vi "Ear control.vi"(11 "Toggle Ears":bool) -> ()   [LabVIEW 2012]
uses:
  <vilib>/Rock Robotics/WPI/Solenoid/WPI_SolenoidValue.ctl
  <vilib>/Rock Robotics/WPI/Solenoid/WPI_SolenoidGetEnum.vi
  <vilib>/Rock Robotics/WPI/Solenoid/WPI_SolenoidSetEnum.vi
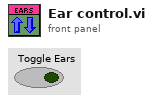
[diagram p1: front panel]
types:
  T1 = typedef "WPI_SolenoidValue.ctl" = enum16{"Off", "On", "Forward", "Reverse"}
  T2 = typedef "WPI_SolenoidDevRef.ctl" = cluster{"DevStatus":errorcluster, "Solenoid Module":T3, "Forward Solenoid Channel":T4, "Reverse Solenoid Channel":T4}
  T3 = typedef "FPGA_TypedefSolenoidModule.ctl" = enum16{"Solenoid Module 1", "Solenoid Module 2"}
  T4 = typedef "WPI_SolenoidChannel.ctl" = enum8{"Solenoid 1", "Solenoid 2", "Solenoid 3", "Solenoid 4", "Solenoid 5", "Solenoid 6", "Solenoid 7", "Solenoid 8", "Invalid"}
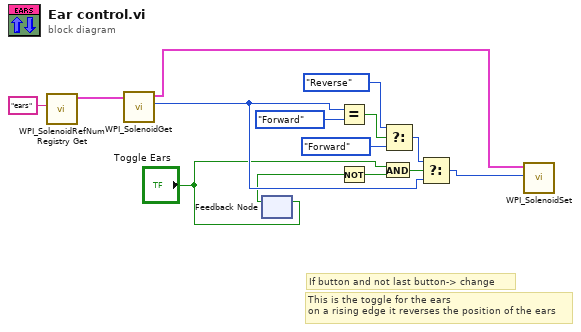
[diagram p0: block diagram]
diagram:
  # "If button and not last button-> change"
  # "This is the toggle for the ears\non a rising edge it reverses the position of the ears"
  n1 = call <vilib>:"WPI_SolenoidRefNum Registry Get.vi"("refnum name"="ears") -> ("SolenoidDevRef"=w7:T2)  [unwired: 9 in, 1 out]
  n2 = call-poly <vilib>:"WPI_SolenoidGet.vi"("SolenoidDevRef"=w7) -> ("Value"=w10:T1, "SolenoidDevRef"=w1:T2)  [unwired: 8 in, 1 out]
  n3 = feedback #1() -> (w5:bool)  [unwired: 1 in]
  n4 = feedback-in #1("Toggle Ears") -> ()
  n5 = Equal?(x=w10, y=WPI_SolenoidValue."Forward" ("s? t:f")) -> (x = y?=w11:bool)
  n6 = Not(x=w5) -> (.not. x?=w3:bool)
  n7 = And(x="Toggle Ears", y=w3) -> (x .and. y?=w6:bool)
  n8 = Select(t=WPI_SolenoidValue."Reverse" ("s? t:f"), s=w11, f=WPI_SolenoidValue."Forward" ("s? t:f")) -> (s? t:f=w14:T1)
  n9 = Select(t=w14, s=w6, f=w10) -> (s? t:f=w2:T1)
  n10 = call-poly <vilib>:"WPI_SolenoidSet.vi"("Value"=w2, "SolenoidDevRef"=w1) -> ()  [unwired: 8 in, 2 out]
